vi "readFromXML.vi"(8 "error in (no error)":errorcluster, 10 "XMLin":string="<guideTargetConfiguration>  \n<target>\n    <raDecParameters>\n      <declination>\n        <degreesDec>0</degreesDec>\n        <minutesArc>0</minutesArc>\n        <secondsArc>0</secondsArc>\n      </declination>\n      <equinoxPrefix>B</equinoxPrefix>\n      <equinoxYear>2000</equinoxYear>\n      <frame>FK4</frame>\n      <ra>\n        <hours>0</hours>\n        <minutesTime>0</minutesTime>\n        <secondsTime>0</secondsTime>\n      </ra>\n    </raDecParameters>\n    <parallax_Arcsec>0</parallax_Arcsec>\n    <properMotion>\n      <epochPM_Yr>2009</epochPM_Yr>\n      <pmdec_ArcsPYr>0</pmdec_ArcsPYr>\n      <pmra_SPYr>0</pmra_SPYr>\n    </properMotion>\n    <rv_kps>0</rv_kps>\n    <targetName></targetName>\n    <difftrack>\n      <dDec_ArcsPS>1</dDec_ArcsPS>\n      <dRA_sps>112.2</dRA_sps>\n    </difftrack>\n  </target>\n  <targetConfigName>this is IT</targetConfigName>  \n  <wl_Microns>0.1</wl_Microns> \n  <commandID>1234</commandID>\n  <tcsErrorResponse>\n   <status>false</status>\n    <code>0</code>\n    <source/>\n  </tcsErrorResponse>\n</guideTargetConfiguration>", 11 "GuideTargetConfiguration in":refnum<class "GuideTargetConfiguration.lvclass">) -> (0 "error out":errorcluster, 3 "GuideTargetConfiguration out":refnum<class "GuideTargetConfiguration.lvclass">)   [LabVIEW 2022 SP3, in "TCSDataDefinitions.lvlib" / "TCSCommand.lvlib" / "TargetConfiguration.lvlib" / "GuideTargetConfiguration.lvclass"]
uses:
  GuideTargetConfiguration.lvclass
  TargetConfiguration/TargetConfiguration.lvclass
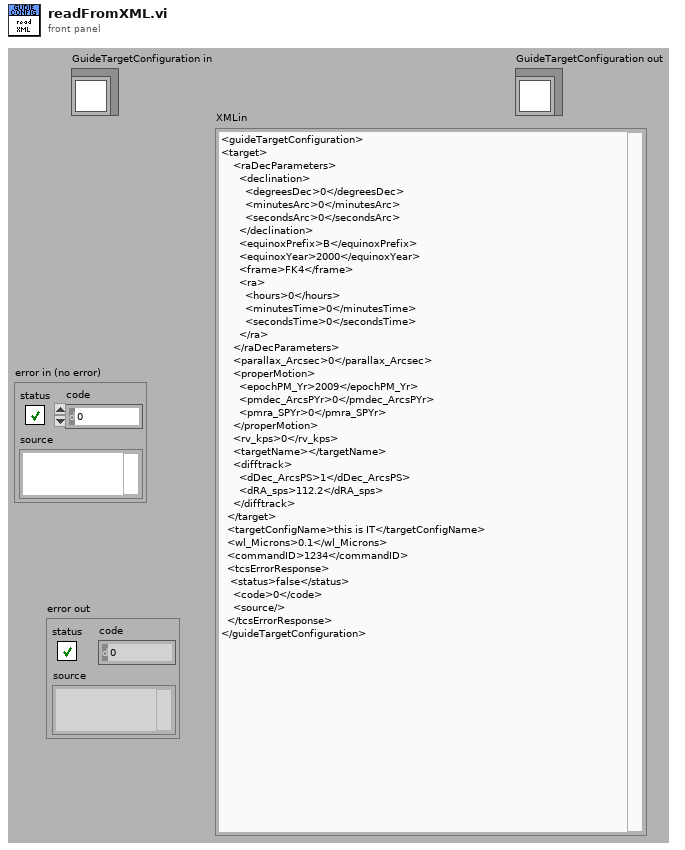
[diagram p1: front panel]
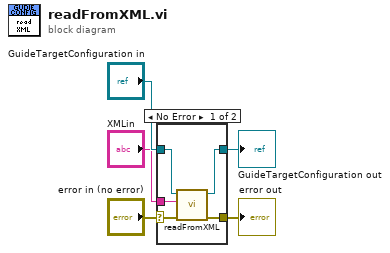
[diagram p0: block diagram]
diagram:
  n1 = case shown="No Error" "error in (no error)" {
    selector: "error in (no error)" -> [w9 w12]
    tunnel: [w8 w12] -> w4
    tunnel: [w6 w11] -> w2
    tunnel: "GuideTargetConfiguration in" -> [w7 w11]
    tunnel: "XMLin" -> [w10 _]
    frame No Error {
      n2 = call-parent "readFromXML.vi"("error in (no error)"=w9, "XMLin"=w10, "TargetConfiguration in"=w7) -> ("error out"=w8:errorcluster, "TargetConfiguration out"=w6:refnum<class "GuideTargetConfiguration.lvclass">)  [unwired: 7 in]
    }
    frame Error {
    }
  }
  "error out" <- w4
  "GuideTargetConfiguration out" <- w2
